vi "JTAG State.vi"(0 "Quick Bit Function (Manual)":T3(ring), 1 "Port (1)":T2(ring), 2 "Value (0)":u8 format="%02x", 3 "Mask (0)":u8 format="%02x", 5 "State (L)":bool, 7 "Function":T1(ring), 11 "error in (no error)":errorcluster) -> (4 "Quick Bit Read":bool, 6 "Manual Read":u8 format="%02x", 15 "error out":errorcluster)   [LabVIEW 2010]
panel:
  # "Manual Inputs"
  # "HIGH"
  # "LOW"
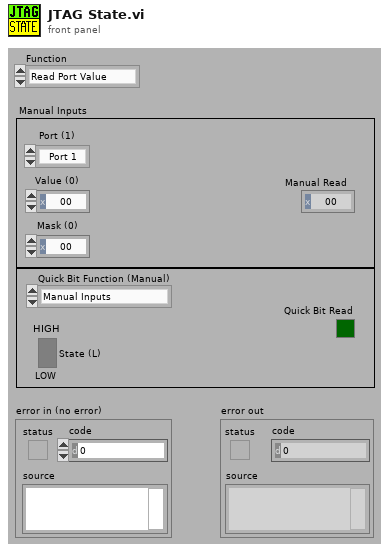
[diagram p1: front panel]
types:
  T1 = enum16{"Read Port Value", "Set Port Value", "Set Port Direction", "Set Port Select", "Set Port Res En"}
  T2 = enum8{"Port 1", "Port 2", "Port 3", "Port 4", "Port 5", "Port 6", "Port 7", "Port 8"}
  T3 = enum16{"Manual Inputs", "PWR_LDO_EN", "PWR_STROBE_IN", "PWR_UV_PROT", "PWR_MAG_TO_OVRD", "PWR_BBC_CTL", "PWR_HVDD_CONN", "<Reserved_1>", "<Reserved_2>", "STIM_RUN", "STIM_STOP", "STIM_CONT", "STIM_SEL", "RST_N", "<Reserved_3>", "TETS_TXD", "<Reserved_4>", "<Reserved_5>", "PWR_MAG_SW (IN)", "PWR_MAG_2S (IN)", "PWR_MAG_5S (IN)", "TETS_RXD (IN)", "PWR_V_DET (IN)", "PWR_BRWN_OUT (IN)", "MICS_IRQ", "<Reserved_7>", "STIM_PROG (IN)", "STIM_PAUSE (IN)", "STIM_SYNC (IN)", "STIM_TFLG (IN)", "STIM_ERR (IN)"}
  T4 = enum16{"Manual Inputs", "PWR_LDO_EN", "PWR_STROBE_IN", "PWR_UV_PROT", "PWR_MAG_TO_OVRD", "PWR_BBC_CTL", "PWR_HVDD_CONN", "<Reserved_1>", "<Reserved_2>", "STIM_RUN", "STIM_STOP", "STIM_CONT", "STIM_SEL", "RST_N", "VHV_SW_ON", "<Reserved_3>", "<Reserved_4>", "<Reserved_5>"}
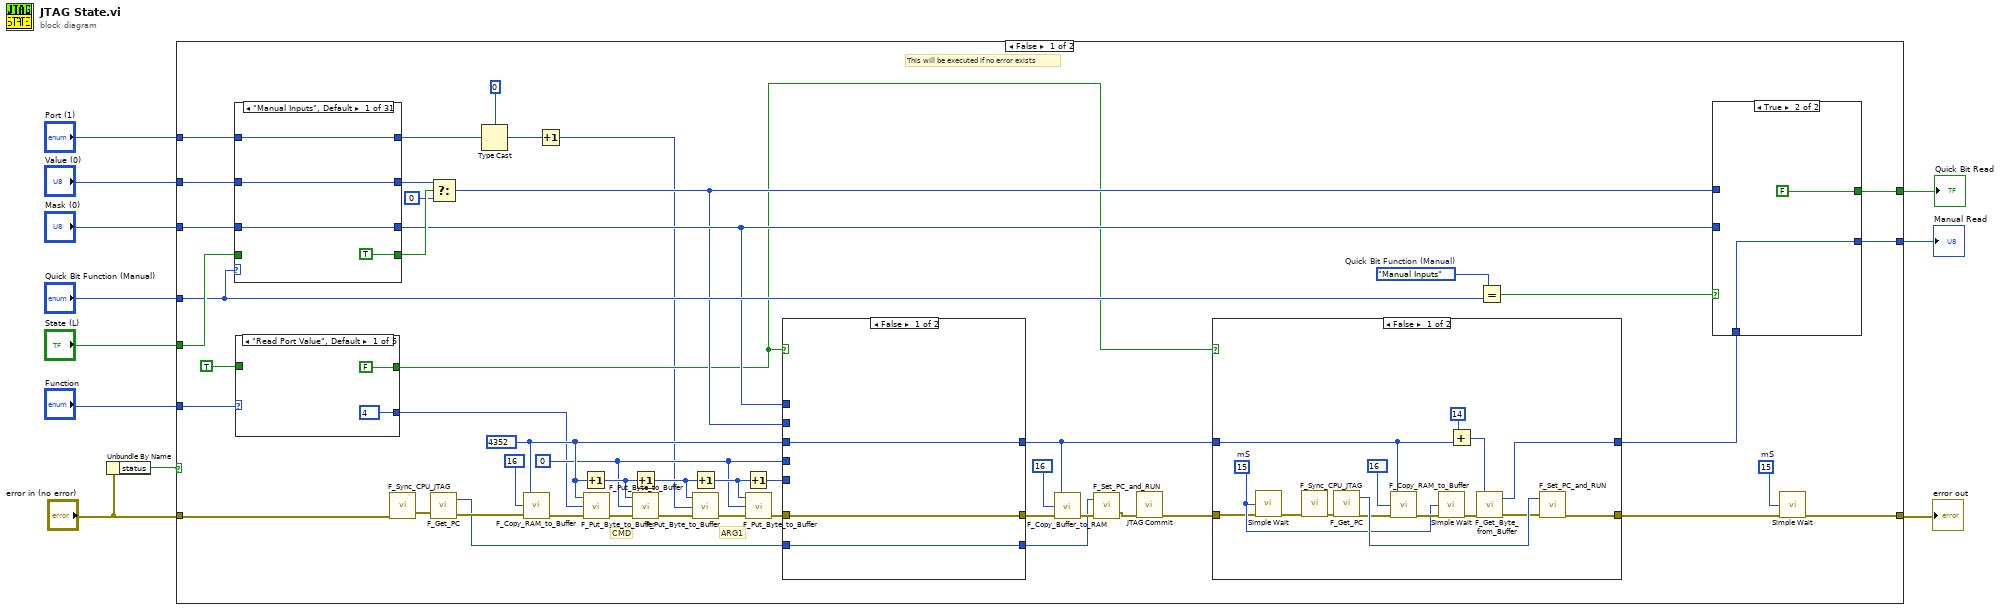
[diagram p0: block diagram]
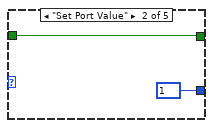
[diagram p2: hidden frame]
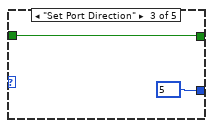
[diagram p3: hidden frame]
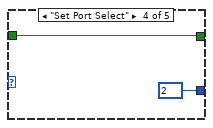
[diagram p4: hidden frame]
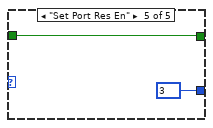
[diagram p5: hidden frame]
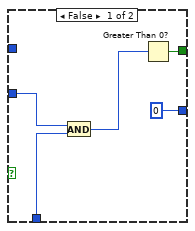
[diagram p6: hidden frame]
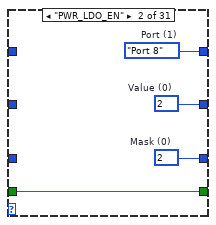
[diagram p7: hidden frame]
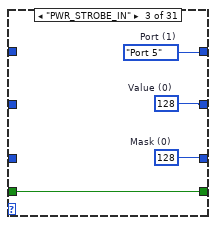
[diagram p8: hidden frame]
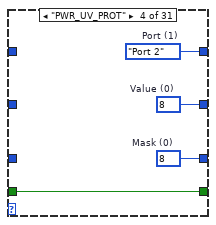
[diagram p9: hidden frame]
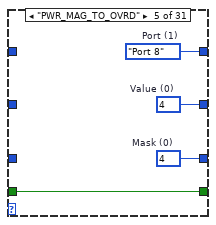
[diagram p10: hidden frame]
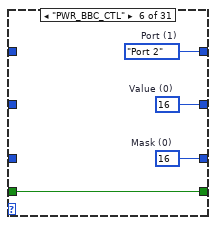
[diagram p11: hidden frame]
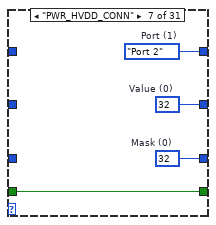
[diagram p12: hidden frame]
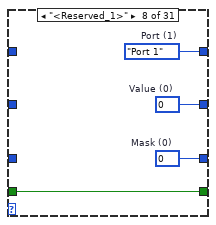
[diagram p13: hidden frame]
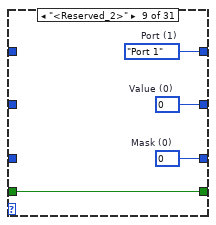
[diagram p14: hidden frame]
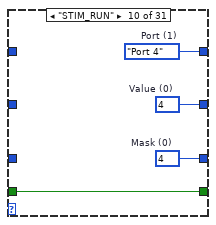
[diagram p15: hidden frame]
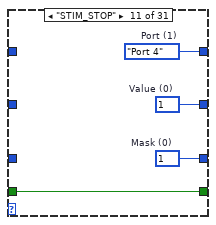
[diagram p16: hidden frame]
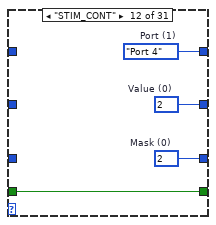
[diagram p17: hidden frame]
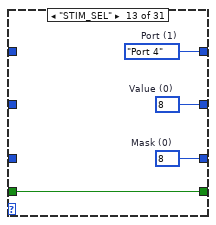
[diagram p18: hidden frame]
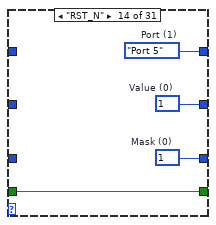
[diagram p19: hidden frame]
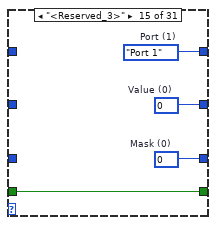
[diagram p20: hidden frame]
diagram:
  n1 = Unbundle By Name("error in (no error)") -> ("status"=w10:bool)
  n2 = case shown="False" w10 {
    tunnel: [w15 w238] -> w11
    tunnel: "error in (no error)" -> [w49 w238]
    tunnel: "Mask (0)" -> [w39 _]
    tunnel: "Value (0)" -> [w40 _]
    tunnel: "Port (1)" -> [w41 _]
    tunnel: "Quick Bit Function (Manual)" -> [w33 _]
    tunnel: "State (L)" -> [w38 _]
    tunnel: "Function" -> [w23 _]
    tunnel: [w32 w236] -> w3
    tunnel: [w31 FALSE] -> w2
    frame False {
      w17 = u32 15  # mS
      w42 = T4."Manual Inputs"  # Quick Bit Function (Manual)
      w50 = u16 4352
      w43 = u16 0
      # "ARG1"
      # "CMD"
      # "This will be executed if no error exists"
      n3 = case shown="\"Manual Inputs\", Default" w33 {
        tunnel: w41 -> [w78 _ _ _ _ _ _ _ _ _ _ _ _ _ _ _ _ _ _ _ _ _ _ _ _ _ _ _ _ _ _]
        tunnel: w40 -> [w81 _ _ _ _ _ _ _ _ _ _ _ _ _ _ _ _ _ _ _ _ _ _ _ _ _ _ _ _ _ _]
        tunnel: w39 -> [w80 _ _ _ _ _ _ _ _ _ _ _ _ _ _ _ _ _ _ _ _ _ _ _ _ _ _ _ _ _ _]
        tunnel: [w78 w84 w87 w91 w95 w98 w102 w109 w110 w116 w121 w125 w129 w131 w137 w138 w145 w149 w151 w156 w161 w163 w168 w173 w177 w178 w185 w189 w193 w197 w201] -> w34
        tunnel: [w81 w83 w88 w92 w96 w99 w103 w108 w111 w117 w120 w124 w128 w133 w136 w141 w144 w148 w153 w157 w160 w165 w169 w172 w176 w179 w184 w188 w192 w196 w200] -> w37
        tunnel: [w80 w82 w89 w93 w97 w101 w104 w107 w112 w115 w119 w123 w127 w132 w135 w140 w143 w147 w152 w155 w159 w164 w167 w171 w175 w181 w183 w187 w191 w195 w199] -> w28
        tunnel: w38 -> [_ w85 w86 w90 w94 w100 w105 w106 w113 w114 w118 w122 w126 w130 w134 w139 w142 w146 w150 w154 w158 w162 w166 w170 w174 w180 w182 w186 w190 w194 w198]
        tunnel: [TRUE ("State (L)") w85 w86 w90 w94 w100 w105 w106 w113 w114 w118 w122 w126 w130 w134 w139 w142 w146 w150 w154 w158 w162 w166 w170 w174 w180 w182 w186 w190 w194 w198] -> w36
        frame "Manual Inputs", Default {
        }
        frame "PWR_LDO_EN" {
          w82 = u8 2  # Mask (0)
          w83 = u8 2  # Value (0)
          w84 = T2."Port 8"  # Port (1)
        }
        frame "PWR_STROBE_IN" {
          w89 = u8 128  # Mask (0)
          w88 = u8 128  # Value (0)
          w87 = T2."Port 5"  # Port (1)
        }
        frame "PWR_UV_PROT" {
          w93 = u8 8  # Mask (0)
          w92 = u8 8  # Value (0)
          w91 = T2."Port 2"  # Port (1)
        }
        frame "PWR_MAG_TO_OVRD" {
          w97 = u8 4  # Mask (0)
          w96 = u8 4  # Value (0)
          w95 = T2."Port 8"  # Port (1)
        }
        frame "PWR_BBC_CTL" {
          w101 = u8 16  # Mask (0)
          w99 = u8 16  # Value (0)
          w98 = T2."Port 2"  # Port (1)
        }
        frame "PWR_HVDD_CONN" {
          w104 = u8 32  # Mask (0)
          w103 = u8 32  # Value (0)
          w102 = T2."Port 2"  # Port (1)
        }
        frame "<Reserved_1>" {
          w107 = u8 0  # Mask (0)
          w108 = u8 0  # Value (0)
          w109 = T2."Port 1"  # Port (1)
        }
        frame "<Reserved_2>" {
          w112 = u8 0  # Mask (0)
          w111 = u8 0  # Value (0)
          w110 = T2."Port 1"  # Port (1)
        }
        frame "STIM_RUN" {
          w115 = u8 4  # Mask (0)
          w117 = u8 4  # Value (0)
          w116 = T2."Port 4"  # Port (1)
        }
        frame "STIM_STOP" {
          w119 = u8 1  # Mask (0)
          w120 = u8 1  # Value (0)
          w121 = T2."Port 4"  # Port (1)
        }
        frame "STIM_CONT" {
          w123 = u8 2  # Mask (0)
          w124 = u8 2  # Value (0)
          w125 = T2."Port 4"  # Port (1)
        }
        frame "STIM_SEL" {
          w127 = u8 8  # Mask (0)
          w128 = u8 8  # Value (0)
          w129 = T2."Port 4"  # Port (1)
        }
        frame "RST_N" {
          w132 = u8 1  # Mask (0)
          w133 = u8 1  # Value (0)
          w131 = T2."Port 5"  # Port (1)
        }
        frame "<Reserved_3>" {
          w135 = u8 0  # Mask (0)
          w136 = u8 0  # Value (0)
          w137 = T2."Port 1"  # Port (1)
        }
        frame "TETS_TXD" {
          w140 = u8 64  # Mask (0)
          w141 = u8 64  # Value (0)
          w138 = T2."Port 3"  # Port (1)
        }
        frame "<Reserved_4>" {
          w143 = u8 0  # Mask (0)
          w144 = u8 0  # Value (0)
          w145 = T2."Port 1"  # Port (1)
        }
        frame "<Reserved_5>" {
          w147 = u8 0  # Mask (0)
          w148 = u8 0  # Value (0)
          w149 = T2."Port 1"  # Port (1)
        }
        frame "PWR_MAG_SW (IN)" {
          w152 = u8 64  # Mask (0)
          w153 = u8 64  # Value (0)
          w151 = T2."Port 1"  # Port (1)
        }
        frame "PWR_MAG_2S (IN)" {
          w155 = u8 1  # Mask (0)
          w157 = u8 1  # Value (0)
          w156 = T2."Port 2"  # Port (1)
        }
        frame "PWR_MAG_5S (IN)" {
          w159 = u8 2  # Mask (0)
          w160 = u8 2  # Value (0)
          w161 = T2."Port 2"  # Port (1)
        }
        frame "TETS_RXD (IN)" {
          w164 = u8 128  # Mask (0)
          w165 = u8 128  # Value (0)
          w163 = T2."Port 3"  # Port (1)
        }
        frame "PWR_V_DET (IN)" {
          w167 = u8 16  # Mask (0)
          w169 = u8 16  # Value (0)
          w168 = T2."Port 1"  # Port (1)
        }
        frame "PWR_BRWN_OUT (IN)" {
          w171 = u8 32  # Mask (0)
          w172 = u8 32  # Value (0)
          w173 = T2."Port 1"  # Port (1)
        }
        frame "MICS_IRQ" {
          w175 = u8 4  # Mask (0)
          w176 = u8 4  # Value (0)
          w177 = T2."Port 1"  # Port (1)
        }
        frame "<Reserved_7>" {
          w181 = u8 0  # Mask (0)
          w179 = u8 0  # Value (0)
          w178 = T2."Port 1"  # Port (1)
        }
        frame "STIM_PROG (IN)" {
          w183 = u8 64  # Mask (0)
          w184 = u8 64  # Value (0)
          w185 = T2."Port 4"  # Port (1)
        }
        frame "STIM_PAUSE (IN)" {
          w187 = u8 32  # Mask (0)
          w188 = u8 32  # Value (0)
          w189 = T2."Port 4"  # Port (1)
        }
        frame "STIM_SYNC (IN)" {
          w191 = u8 16  # Mask (0)
          w192 = u8 16  # Value (0)
          w193 = T2."Port 4"  # Port (1)
        }
        frame "STIM_TFLG (IN)" {
          w195 = u8 64  # Mask (0)
          w196 = u8 64  # Value (0)
          w197 = T2."Port 2"  # Port (1)
        }
        frame "STIM_ERR (IN)" {
          w199 = u8 128  # Mask (0)
          w200 = u8 128  # Value (0)
          w201 = T2."Port 2"  # Port (1)
        }
      }
      n4 = case shown="\"Read Port Value\", Default" w23 {
        tunnel: [u8 4 ("Value (0)") u8 1 ("Value (0)") u8 5 ("Value (0)") u8 2 ("Value (0)") u8 3 ("Value (0)")] -> w22
        tunnel: [FALSE w63 w65 w67 w69] -> w21
        tunnel: TRUE -> [_ w63 w65 w67 w69]
        frame "Read Port Value", Default {
        }
        frame "Set Port Value" {
        }
        frame "Set Port Direction" {
        }
        frame "Set Port Select" {
        }
        frame "Set Port Res En" {
        }
      }
      n5 = call "F_Sync_CPU_JTAG.vi"("error in (no error)"=w49) -> ("error out"=w26:errorcluster)  [unwired: 1 in, 1 out]
      n6 = Select(t=w37, s=w36, f=u8 0) -> (s? t:f=w27:u8)
      n7 = call "F_Get_PC.vi"("error in (no error)"=w26) -> ("error out"=w25:errorcluster, "Program Counter"=w24:u16)  [unwired: 1 in]
      n8 = Type Cast(type=u8 0, x=w34) -> (*(type *) &x=w13:u8)
      n9 = call "F_Copy_RAM_to_Buffer.vi"("error in (no error)"=w25, "Block size to be copied"=u16 16, "RAM start address"=w50) -> ("error out"=w58:errorcluster)  [unwired: 2 in]
      n10 = Increment(x=w13) -> (x+1=w14:u8)
      n11 = Increment(x=w50) -> (x+1=w59:u16)
      n12 = call "F_Put_Byte_to_Buffer.vi"("error in (no error)"=w58, "New value"=w22, "Address of byte to be updated"=w50) -> ("error out"=w60:errorcluster)  [unwired: 2 in]
      n13 = Increment(x=w59) -> (x+1=w54:u16)
      n14 = call "F_Put_Byte_to_Buffer.vi"("error in (no error)"=w60, "New value"=w43, "Address of byte to be updated"=w59) -> ("error out"=w51:errorcluster)  [unwired: 2 in]
      n15 = Increment(x=w54) -> (x+1=w55:u16)
      n16 = call "F_Put_Byte_to_Buffer.vi"("error in (no error)"=w51, "New value"=w14, "Address of byte to be updated"=w54) -> ("error out"=w56:errorcluster)  [unwired: 2 in]
      n17 = Increment(x=w55) -> (x+1=w53:u16)
      n18 = call "F_Put_Byte_to_Buffer.vi"("error in (no error)"=w56, "New value"=w43, "Address of byte to be updated"=w55) -> ("error out"=w52:errorcluster)  [unwired: 2 in]
      n19 = case shown="False" w21 {
        tunnel: w53 -> [_ w229]
        tunnel: w52 -> [w221 w228]
        tunnel: w24 -> [w220 w226]
        tunnel: w43 -> [_ w224]
        tunnel: w50 -> [w219 w227]
        tunnel: [w219 w227] -> w44
        tunnel: [w220 w226] -> w45
        tunnel: [w221 w225] -> w46
        tunnel: w27 -> [_ w223]
        tunnel: w28 -> [_ w222]
        frame False {
        }
        frame True {
          # "ARG2"
          # "ARG3"
          n20 = Increment(x=w229) -> (x+1=w234:u16)
          n21 = call "F_Put_Byte_to_Buffer.vi"("error in (no error)"=w228, "New value"=w223, "Address of byte to be updated"=w229) -> ("error out"=w235:errorcluster)  [unwired: 2 in]
          n22 = Increment(x=w234) -> (x+1=w230:u16)
          n23 = call "F_Put_Byte_to_Buffer.vi"("error in (no error)"=w235, "New value"=w224, "Address of byte to be updated"=w234) -> ("error out"=w231:errorcluster)  [unwired: 2 in]
          n24 = call "F_Put_Byte_to_Buffer.vi"("error in (no error)"=w231, "New value"=w222, "Address of byte to be updated"=w230) -> ("error out"=w233:errorcluster)  [unwired: 2 in]
          n25 = Increment(x=w230) -> (x+1=w232:u16)
          n26 = call "F_Put_Byte_to_Buffer.vi"("error in (no error)"=w233, "New value"=w224, "Address of byte to be updated"=w232) -> ("error out"=w225:errorcluster)  [unwired: 2 in]
        }
      }
      n27 = call "F_Copy_Buffer_to_RAM.vi"("error in (no error)"=w46, "Block size to be copied"=u16 16, "Buffer start address"=w44) -> ("error out"=w48:errorcluster)  [unwired: 2 in]
      n28 = call "F_Set_PC_and_RUN.vi"("error in (no error)"=w48, "PC start address"=w45) -> ("error out"=w19:errorcluster)  [unwired: 1 in]
      n29 = call "JTAG Commit.vi"("error in (no error)"=w19) -> ("error out"=w18:errorcluster)  [unwired: 10 in]
      n30 = case shown="False" w21 {
        tunnel: w18 -> [w203 w217]
        tunnel: w44 -> [w205 _]
        tunnel: [w204 u16 0] -> w30
        tunnel: [w202 w217] -> w16
        frame False {
          w211 = u32 15  # mS
          n31 = call "Simple Wait.vi"("mS"=w211, "error in"=w203) -> ("error out"=w209:errorcluster)  [unwired: 12 in, 1 out]
          n32 = call "F_Sync_CPU_JTAG.vi"("error in (no error)"=w209) -> ("error out"=w215:errorcluster)  [unwired: 1 in, 1 out]
          n33 = call "F_Get_PC.vi"("error in (no error)"=w215) -> ("error out"=w214:errorcluster, "Program Counter"=w216:u16)  [unwired: 1 in]
          n34 = call "F_Copy_RAM_to_Buffer.vi"("error in (no error)"=w214, "Block size to be copied"=16, "RAM start address"=w205) -> ("error out"=w212:errorcluster)  [unwired: 2 in]
          n35 = call "Simple Wait.vi"("mS"=w211, "error in"=w212) -> ("error out"=w213:errorcluster)  [unwired: 12 in, 1 out]
          n36 = Add(x=14 ("Block size to be copied"), y=w205) -> (x+y=w207:i32)
          n37 = call "F_Get_Byte_from_Buffer.vi"("error in (no error)"=w213, "Address of byte to be read"=w207) -> ("error out"=w208:errorcluster, "Current value"=w204:u8)
          n38 = call "F_Set_PC_and_RUN.vi"("error in (no error)"=w208, "PC start address"=w216) -> ("error out"=w202:errorcluster)  [unwired: 1 in]
        }
        frame True {
        }
      }
      n39 = Equal?(x=w42, y=w33) -> (x = y?=w29:bool)
      n40 = case shown="True" w29 {
        tunnel: [0 w77] -> w32
        tunnel: [w72 FALSE] -> w31
        tunnel: w30 -> [w74 w77]
        tunnel: w28 -> [w73 _]
        tunnel: w27 -> [_ _]
        frame False {
          n41 = And(x=w73, y=w74) -> (x .and. y?=w71:u16)
          n42 = Greater Than 0?(x=w71) -> (x > 0?=w72:bool)
        }
        frame True {
        }
      }
      n43 = call "Simple Wait.vi"("mS"=w17, "error in"=w16) -> ("error out"=w15:errorcluster)  [unwired: 12 in, 1 out]
    }
    frame True {
      w236 = 0  # Current value
      # "Error exists, skip all functions"
    }
  }
  "error out" <- w11
  "Quick Bit Read" <- w2
  "Manual Read" <- w3
